vi "GetNet-Client Check Network Parameters.vi"(8 "error in (no error)":errorcluster, 9 "Timeout":i32, 10 "Port":u16, 11 "IP":string) -> (0 "error out":errorcluster)   [LabVIEW 2014, in "GenNet-Client.lvlib"]
doc: "Checks the connection parameters for valid settings (IP address, port number)"
uses:
  GenNet-Client.lvlib
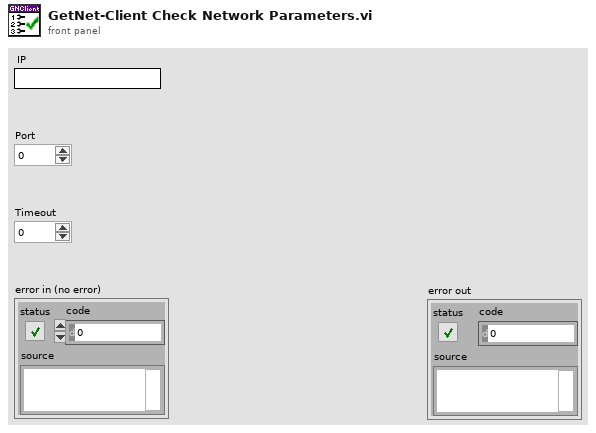
[diagram p1: front panel]
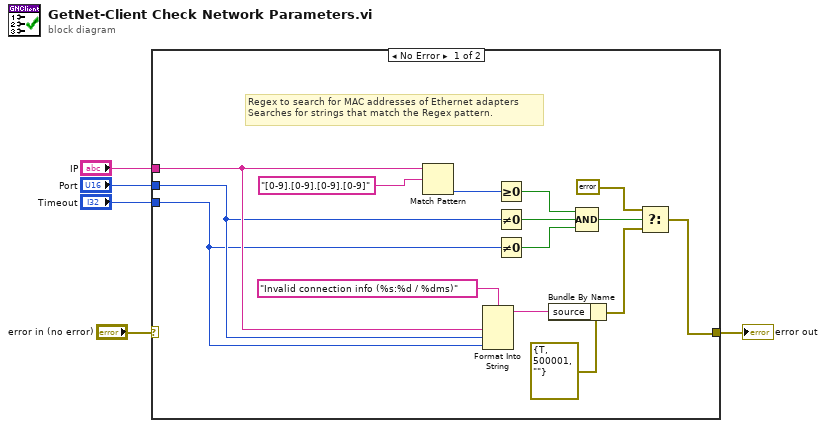
[diagram p0: block diagram]
diagram:
  n1 = case shown="No Error" "error in (no error)" {
    selector: "error in (no error)" -> [_ w21]
    tunnel: [w14 w21] -> w4
    tunnel: "IP" -> [w9 _]
    tunnel: "Port" -> [w8 _]
    tunnel: "Timeout" -> [w6 _]
    frame No Error {
      # "Regex to search for MAC addresses of Ethernet adapters\nSearches for strings that match the Regex pattern."
      n2 = Match Pattern(string=w9, regular expression="[0-9].[0-9].[0-9].[0-9]") -> (offset past match=w19:i32)  [unwired: 1 in, 3 out]
      n3 = Format Into String(format string="Invalid connection info (%s:%d / %dms)", w9, w8, w6) -> (resulting string=w10:string)  [unwired: 2 in, 1 out]
      n4 = Greater Or Equal To 0?(x=w19) -> (x >= 0?=w18:bool)
      n5 = Not Equal To 0?(x=w8) -> (x != 0?=w17:bool)
      n6 = Not Equal To 0?(x=w6) -> (x != 0?=w7:bool)
      n7 = Bundle By Name(cluster=errorcluster {"status"=TRUE, "code"=500001, "source"=""} ("error IO"), "source"=w10) -> (w12:errorcluster)
      n8 = Compound Arithmetic op=AND(w18, w17, w7) -> (w16:bool)
      n9 = Select(t=errorcluster {"status"=FALSE, "code"=0, "source"=""} ("error IO"), s=w16, f=w12) -> (s? t:f=w14:errorcluster)
    }
    frame Error {
    }
  }
  "error out" <- w4
